vi "calculate_max_abs_from_equal.vi"(8 "error in (no error)":errorcluster, 10 "String":string, 11 "MAX":string) -> (0 "error out":errorcluster, 3 "MAX":dbl)   [LabVIEW 2017]
uses:
  <vilib>/gmath/NI_Gmath.lvlib
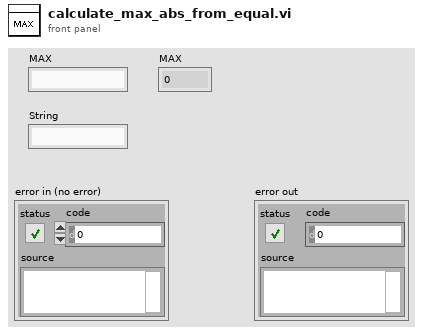
[diagram p1: front panel]
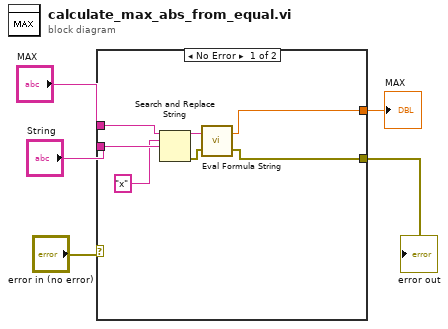
[diagram p0: block diagram]
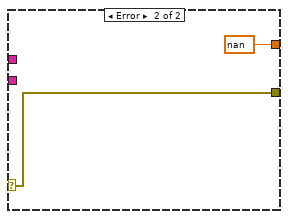
[diagram p2: hidden frame]
diagram:
  n1 = case shown="No Error" "error in (no error)" {
    selector: "error in (no error)" -> [_ w14]
    tunnel: [w12 nan ("y value")] -> w5
    tunnel: "String" -> [w11 _]
    tunnel: "MAX" -> [w9 _]
    tunnel: [w6 w14] -> w2
    frame No Error {
      n2 = Search and Replace String(input string=w9, search string="x", replace string=w11) -> (result string=w8:string, error out=w7:errorcluster)  [unwired: 5 in, 2 out]
      n3 = call <vilib>:"Eval Formula String.vi"("error in (no error)"=w7, "formula"=w8) -> ("error out"=w6:errorcluster, "y value"=w12:dbl)
    }
    frame Error {
    }
  }
  "MAX" <- w5
  "error out" <- w2
